vi "automat.vi"() -> ()   [LabVIEW 2014]
uses:
  Timer 2013/Control Timer.ctl
  <vilib>/functionblocks/Edge Detection/One Shot Falling With Input/One Shot Falling With Input.vi
  <vilib>/functionblocks/Edge Detection/One Shot Rising with Input/One Shot Rising with Input.vi
  <vilib>/functionblocks/FB Core/FB Core.xnode
  <vilib>/functionblocks/NI_FunctionBlock Libraries.lvlib
panel:
  out "Center":dbl
  out "Enum 2":T1(ring)
  out "Shutdown":dbl
  out "Left":dbl
  out "Right":dbl
  out "Fault":bool
  out "Right":bool
  out "Center":bool
  out "Left":bool
  in  "Enum":T1(ring)
  out "error out":errorcluster
  in  "error in (no error)":errorcluster
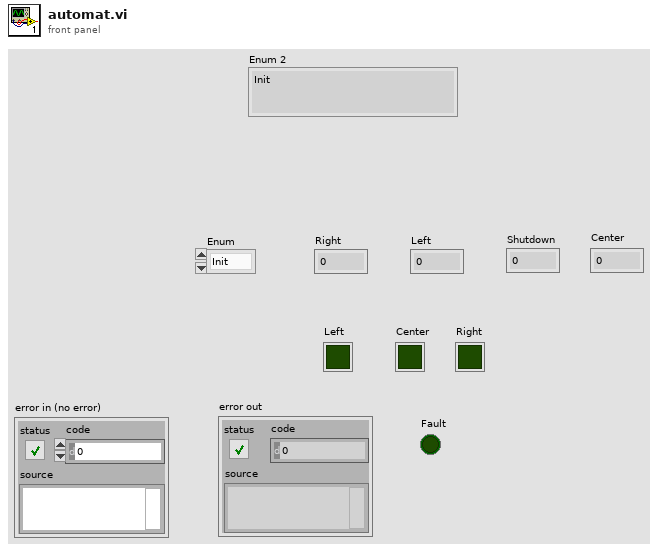
[diagram p1: front panel]
types:
  T1 = enum16{"Init", "Ready", "Shutdown", "Left", "Center", "Right", "Powering up", "Emergency", "Powering down"}
  T2 = typedef "Control Timer.ctl" = enum16{"Timecheck", "Reset"}
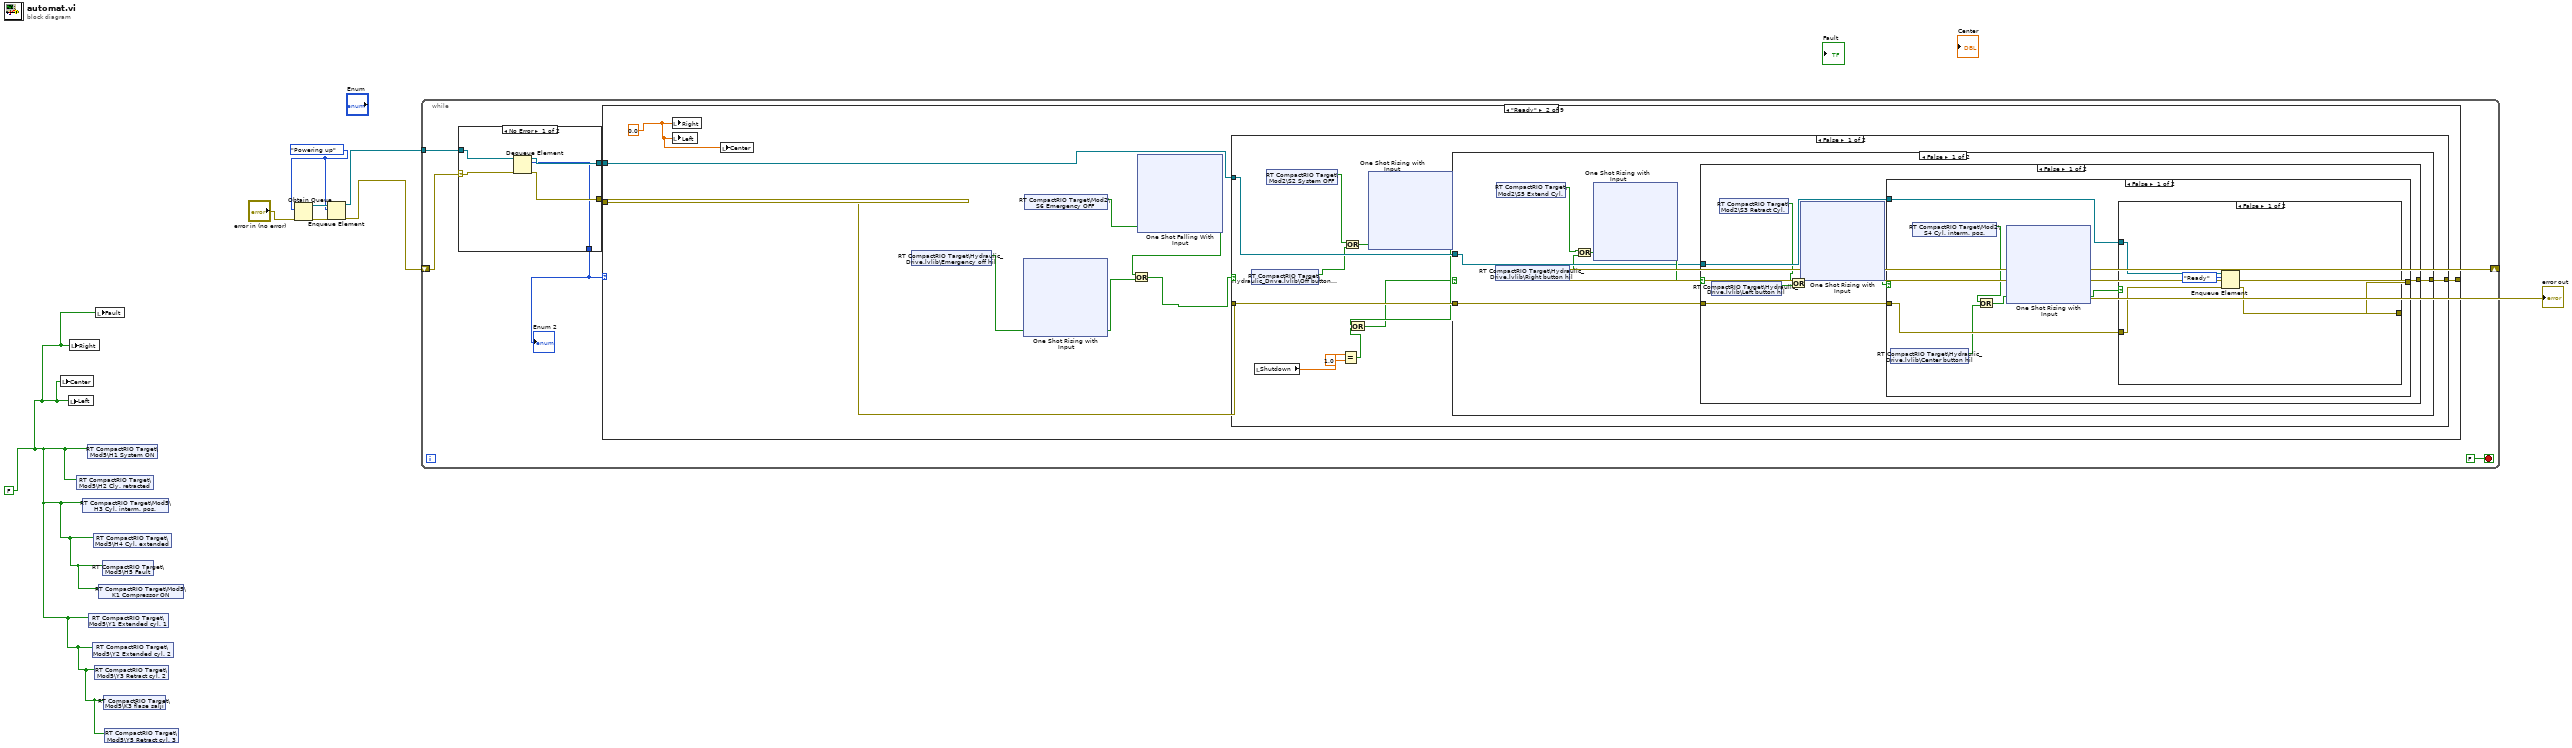
[diagram p0: block diagram]
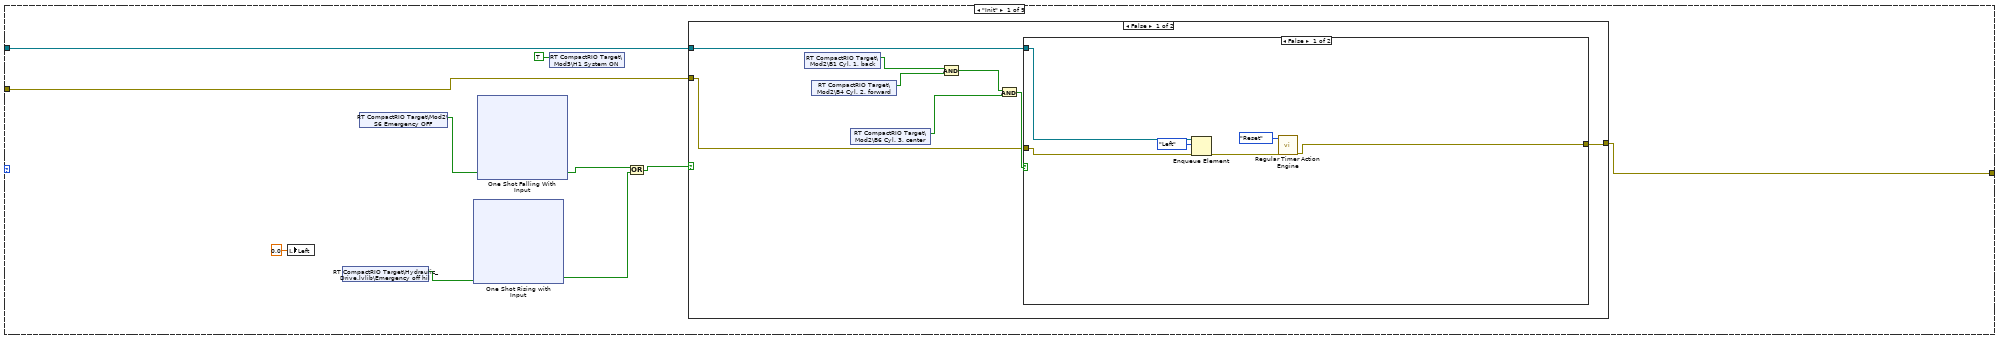
[diagram p2: hidden frame]
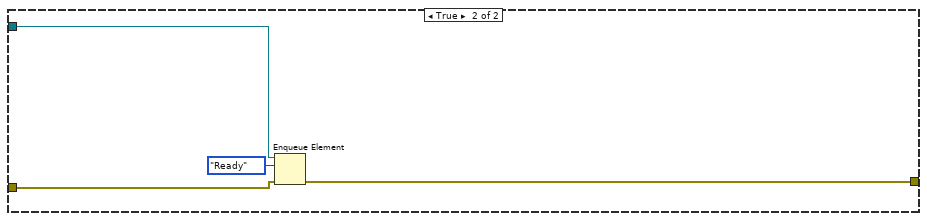
[diagram p3: hidden frame]
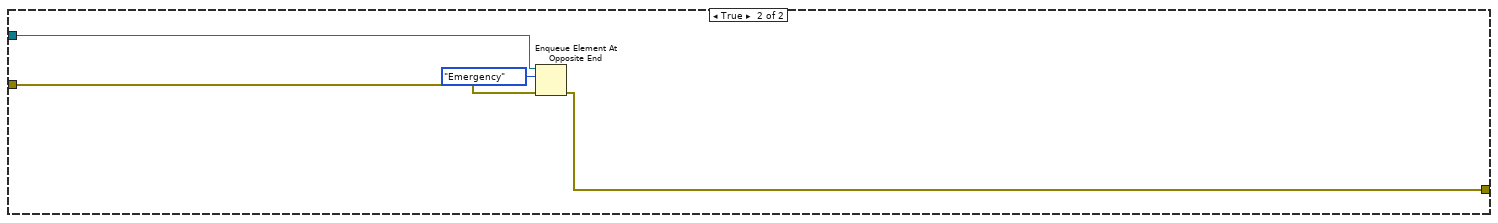
[diagram p4: hidden frame]
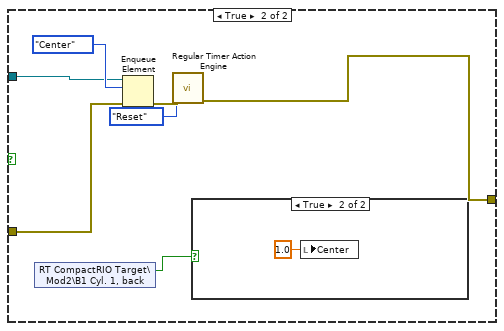
[diagram p5: hidden frame]
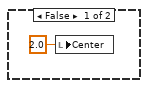
[diagram p6: hidden frame]
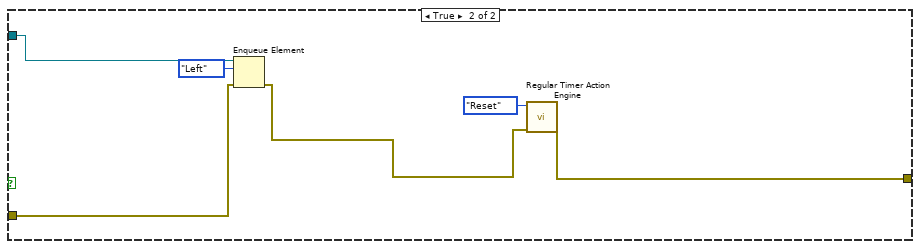
[diagram p7: hidden frame]
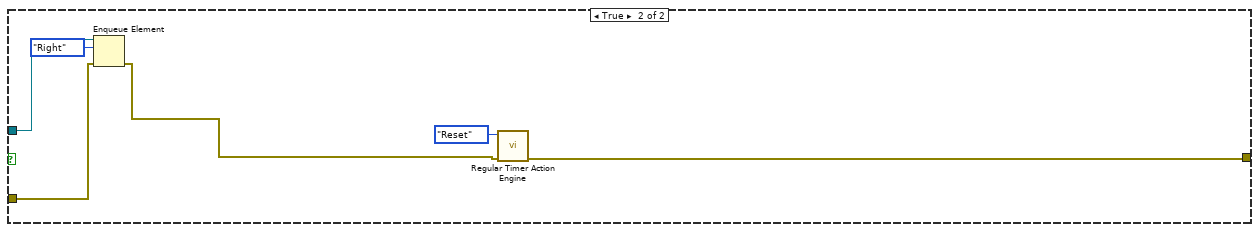
[diagram p8: hidden frame]
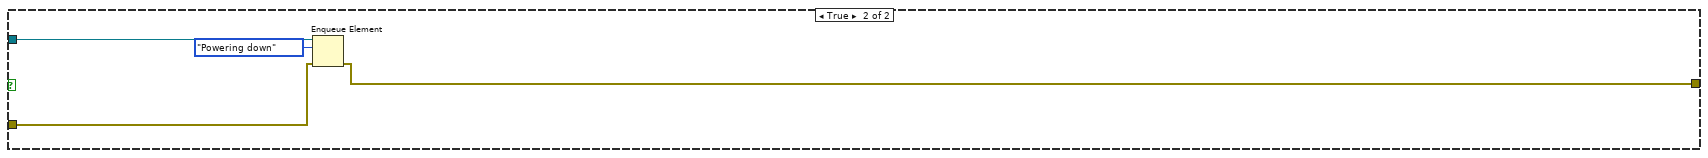
[diagram p9: hidden frame]
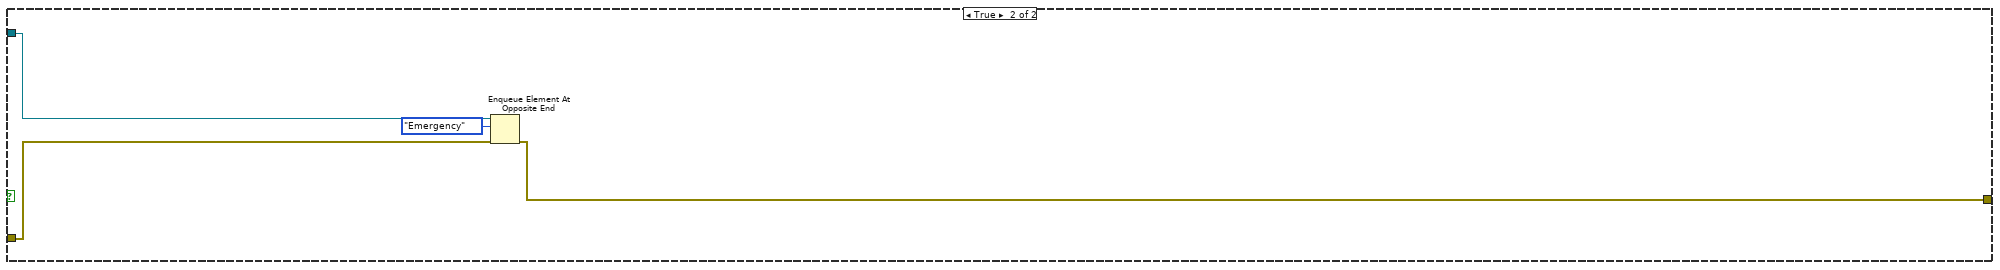
[diagram p10: hidden frame]
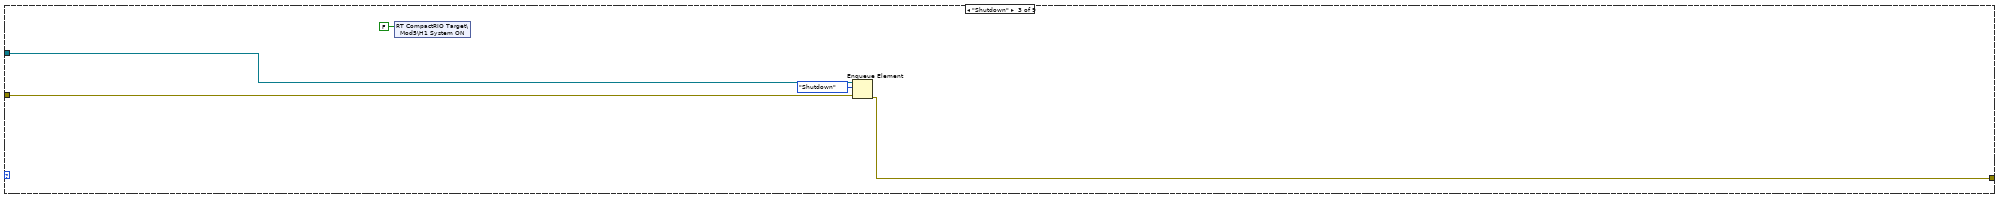
[diagram p11: hidden frame]
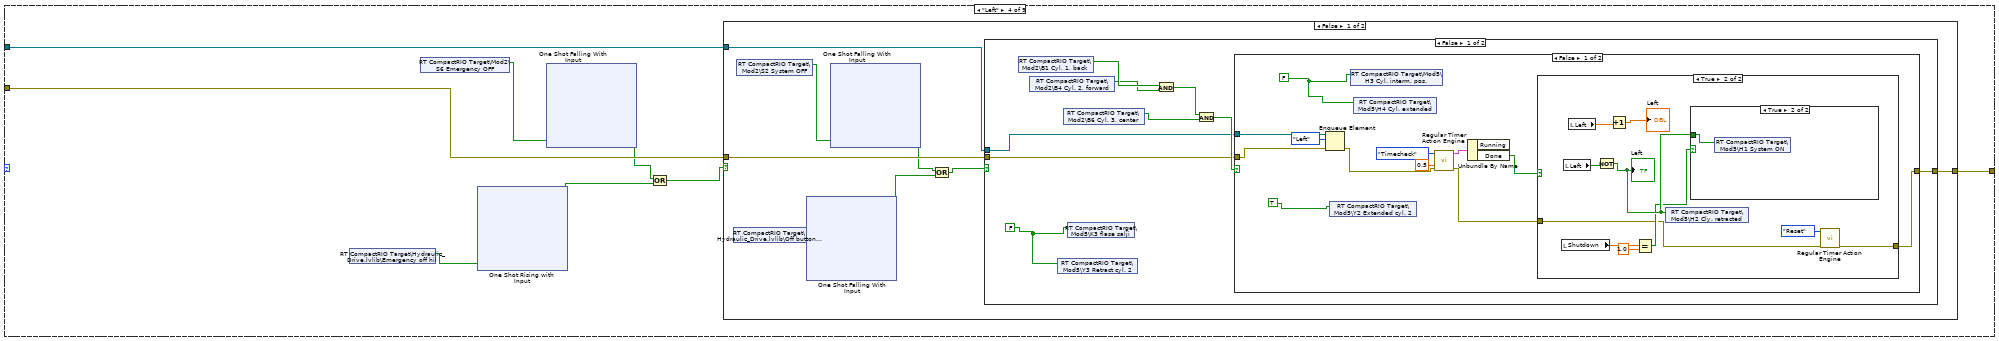
[diagram p12: hidden frame]
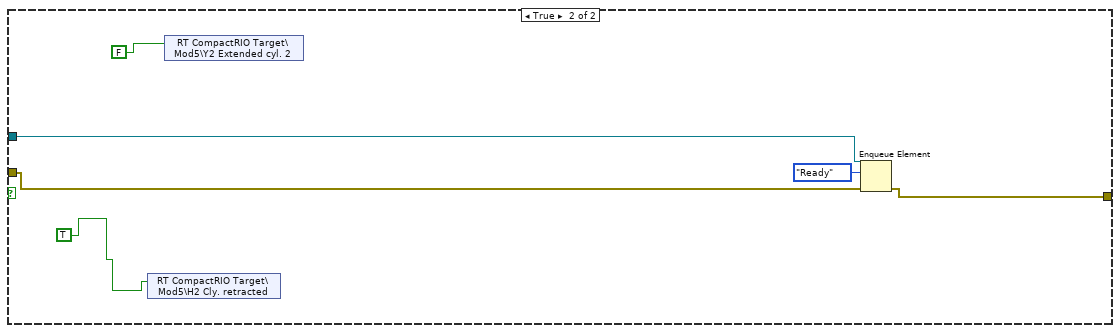
[diagram p15: hidden frame]
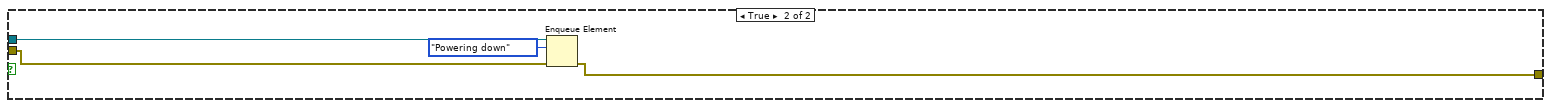
[diagram p16: hidden frame]
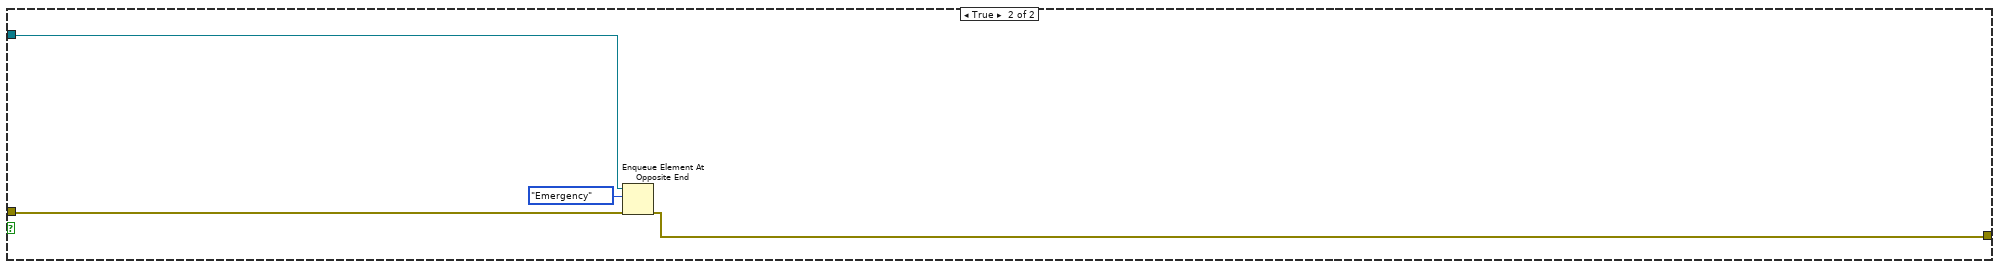
[diagram p17: hidden frame]
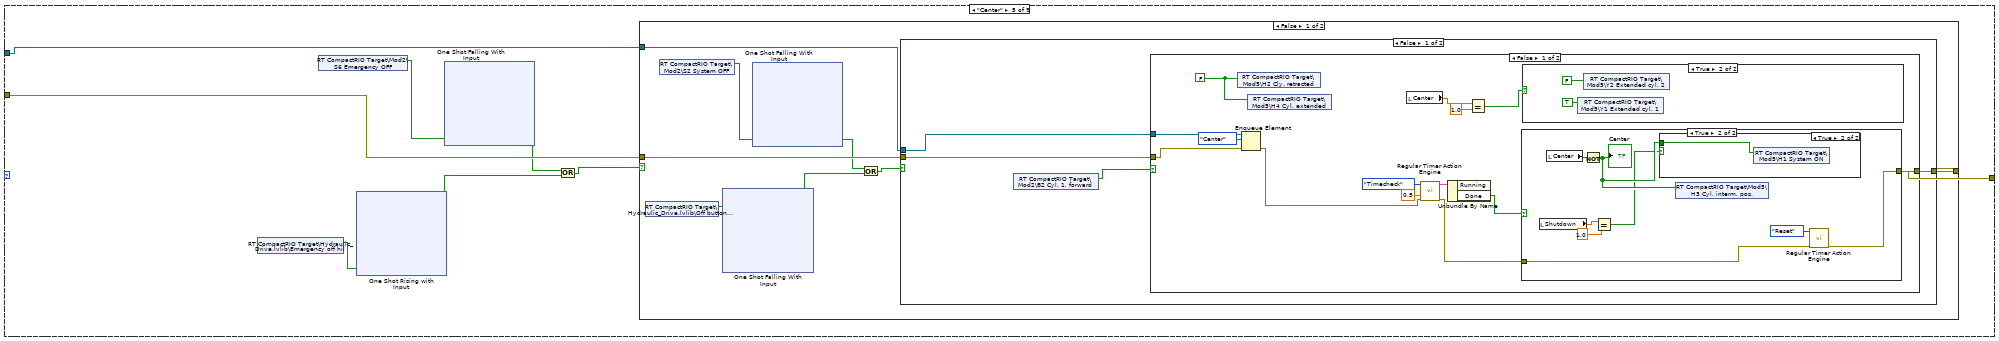
[diagram p18: hidden frame]
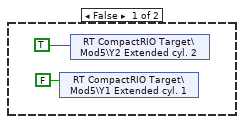
[diagram p19: hidden frame]
diagram:
  w1 = FALSE
  w5 = T1."Powering up" ("Enum")
  n1 = local write "Center"(w1) -> ()
  n2 = local write "Left"(w1) -> ()
  n3 = local write "Right"(w1) -> ()
  n4 = shared-variable "RT CompactRIO Target\\Mod5\\H2 Cly. retracted"(w1) -> ()  [unwired: 1 in, 1 out]
  n5 = shared-variable "RT CompactRIO Target\\Mod5\\H3 Cyl. interm. pos."(w1) -> ()  [unwired: 1 in, 1 out]
  n6 = shared-variable "RT CompactRIO Target\\Mod5\\H1 System ON"(w1) -> ()  [unwired: 1 in, 1 out]
  n7 = shared-variable "RT CompactRIO Target\\Mod5\\Y1 Extended cyl. 1"(w1) -> ()  [unwired: 1 in, 1 out]
  n8 = shared-variable "RT CompactRIO Target\\Mod5\\Y2 Extended cyl. 2"(w1) -> ()  [unwired: 1 in, 1 out]
  n9 = shared-variable "RT CompactRIO Target\\Mod5\\H4 Cyl. extended"(w1) -> ()  [unwired: 1 in, 1 out]
  n10 = shared-variable "RT CompactRIO Target\\Mod5\\Y3 Retract cyl. 2"(w1) -> ()  [unwired: 1 in, 1 out]
  n11 = local write "Fault"(w1) -> ()
  n12 = shared-variable "RT CompactRIO Target\\Mod5\\K1 Compressor ON"(w1) -> ()  [unwired: 1 in, 1 out]
  n13 = shared-variable "RT CompactRIO Target\\Mod5\\H5 Fault"(w1) -> ()  [unwired: 1 in, 1 out]
  n14 = shared-variable "RT CompactRIO Target\\Mod5\\K3 flase salji"(w1) -> ()  [unwired: 1 in, 1 out]
  n15 = shared-variable "RT CompactRIO Target\\Mod5\\Y5 Retract cyl. 3"(w1) -> ()  [unwired: 1 in, 1 out]
  n16 = Obtain Queue(element data type=w5, error in (no error)="error in (no error)") -> (queue out=w6:refnum<queue>, error out=w7:errorcluster)  [unwired: 3 in, 1 out]
  n17 = Enqueue Element(queue=w6, element=w5, error in (no error)=w7) -> (queue out=w4:refnum<queue>, error out=w2:errorcluster)  [unwired: 1 in, 1 out]
  n18 = while {
    tunnel: w4 -> [w15]
    shift-right: [w12] -> w3
    shift-left: w2 -> [w11]
    stop <- FALSE stop-if-true
    n19 = case shown="No Error" w11 {
      selector: w11 -> [w1333 w1336]
      tunnel: w15 -> [w1331 w1335]
      tunnel: [w1332 w1336] -> w13
      tunnel: [w1330 w1335] -> w14
      tunnel: [w1329 T1."Shutdown" ("Enum")] -> w9
      frame No Error {
        n20 = Dequeue Element(queue=w1331, error in (no error)=w1333) -> (queue out=w1330:refnum<queue>, element=w1329:T1, error out=w1332:errorcluster)  [unwired: 1 in, 1 out]
      }
      frame Error {
      }
    }
    "Enum 2" <- w9
    n21 = case shown="\"Ready\"" w9 {
      tunnel: w14 -> [w22 w131 w428 w436 w650 w865 w1080 w1238 w1327]
      tunnel: w13 -> [w23 w132 w429 w437 w651 w866 w1081 w1237 w1328]
      tunnel: [w21 w130 w427 w435 w652 w864 w1079 w1232 w1325] -> w12
      frame "Init" {
        n22 = local write "Left"(0.0 ("Left")) -> ()
        n23 = shared-variable "RT CompactRIO Target\\Hydraulic_Drive.lvlib\\Emergency off hil"() -> (w16:bool)  [unwired: 1 in, 1 out]
        n24 = shared-variable "RT CompactRIO Target\\Mod2\\S6 Emergency OFF"() -> (w24:bool)  [unwired: 1 in, 1 out]
        n25 = xnode "One Shot Rising with Input"("input"=w16) -> ("output"=w17:bool)  [unwired: 1 in, 1 out]
        n26 = xnode "One Shot Falling With Input"("input"=w24) -> ("output"=w18:bool)  [unwired: 1 in, 1 out]
        n27 = shared-variable "RT CompactRIO Target\\Mod5\\H1 System ON"(TRUE ("H1 System ON")) -> ()  [unwired: 1 in, 1 out]
        n28 = Or(x=w18, y=w17) -> (x .or. y?=w19:bool)
        n29 = case shown="False" w19 {
          tunnel: w23 -> [w66 w85]
          tunnel: w22 -> [w64 w84]
          tunnel: [w65 w82] -> w21
          frame False {
            n30 = shared-variable "RT CompactRIO Target\\Mod2\\B1 Cyl. 1, back"() -> (w71:bool)  [unwired: 1 in, 1 out]
            n31 = shared-variable "RT CompactRIO Target\\Mod2\\B4 Cyl. 2, forward"() -> (w70:bool)  [unwired: 1 in, 1 out]
            n32 = shared-variable "RT CompactRIO Target\\Mod2\\B6 Cyl. 3, center"() -> (w68:bool)  [unwired: 1 in, 1 out]
            n33 = And(x=w71, y=w70) -> (x .and. y?=w69:bool)
            n34 = And(x=w69, y=w68) -> (x .and. y?=w67:bool)
            n35 = case shown="False" w67 {
              tunnel: w66 -> [w77 w81]
              tunnel: [w73 w80] -> w65
              tunnel: w64 -> [w76 w79]
              frame False {
                n36 = Enqueue Element(queue=w76, element=T1."Left", error in (no error)=w77) -> (error out=w74:errorcluster)  [unwired: 1 in, 2 out]
                n37 = call "Regular Timer Action Engine.vi"("Enum"=Control_Timer."Reset", "error in"=w74) -> ("error out"=w73:errorcluster)  [unwired: 7 in, 1 out]
              }
              frame True {
                n38 = Enqueue Element(queue=w79, element=T1."Ready", error in (no error)=w81) -> (error out=w80:errorcluster)  [unwired: 1 in, 2 out]
              }
            }
          }
          frame True {
            n39 = Enqueue Element At Opposite End(queue=w84, element=T1."Emergency", error in (no error)=w85) -> (error out=w82:errorcluster)  [unwired: 1 in, 2 out]
          }
        }
      }
      frame "Ready" {
        w125 = 0.0
        n40 = local write "Right"(w125) -> ()
        n41 = local write "Left"(w125) -> ()
        n42 = local write "Center"(w125) -> ()
        n43 = shared-variable "RT CompactRIO Target\\Hydraulic_Drive.lvlib\\Emergency off hil"() -> (w129:bool)  [unwired: 1 in, 1 out]
        n44 = xnode "One Shot Rising with Input"("input"=w129) -> ("output"=w128:bool)  [unwired: 1 in, 1 out]
        n45 = shared-variable "RT CompactRIO Target\\Mod2\\S6 Emergency OFF"() -> (w127:bool)  [unwired: 1 in, 1 out]
        n46 = xnode "One Shot Falling With Input"("input"=w127) -> ("output"=w126:bool)  [unwired: 1 in, 1 out]
        n47 = Or(x=w126, y=w128) -> (x .or. y?=w124:bool)
        n48 = case shown="False" w124 {
          tunnel: w132 -> [w181 w387]
          tunnel: w131 -> [w179 w386]
          tunnel: [w180 w384] -> w130
          frame False {
            n49 = shared-variable "RT CompactRIO Target\\Hydraulic_Drive.lvlib\\Off button hil"() -> (w176:bool)  [unwired: 1 in, 1 out]
            n50 = local read "Shutdown"() -> (w173:dbl)
            n51 = shared-variable "RT CompactRIO Target\\Mod2\\S2 System OFF"() -> (w177:bool)  [unwired: 1 in, 1 out]
            n52 = Equal?(x=w173, y=1.0) -> (x = y?=w175:bool)
            n53 = Or(x=w177, y=w176) -> (x .or. y?=w178:bool)
            n54 = xnode "One Shot Rising with Input"("input"=w178) -> ("output"=w172:bool)  [unwired: 1 in, 1 out]
            n55 = Or(x=w172, y=w175) -> (x .or. y?=w171:bool)
            n56 = case shown="False" w171 {
              tunnel: w181 -> [w225 w383]
              tunnel: [w223 w382] -> w180
              tunnel: w179 -> [w224 w381]
              frame False {
                n57 = shared-variable "RT CompactRIO Target\\Hydraulic_Drive.lvlib\\Right button hil"() -> (w220:bool)  [unwired: 1 in, 1 out]
                n58 = shared-variable "RT CompactRIO Target\\Mod2\\S5 Extend Cyl."() -> (w221:bool)  [unwired: 1 in, 1 out]
                n59 = Or(x=w221, y=w220) -> (x .or. y?=w222:bool)
                n60 = xnode "One Shot Rising with Input"("input"=w222) -> ("output"=w226:bool)  [unwired: 1 in, 1 out]
                n61 = case shown="False" w226 {
                  tunnel: w225 -> [w232 w341]
                  tunnel: w224 -> [w231 w340]
                  tunnel: [w230 w336] -> w223
                  frame False {
                    n62 = shared-variable "RT CompactRIO Target\\Hydraulic_Drive.lvlib\\Left button hil"() -> (w227:bool)  [unwired: 1 in, 1 out]
                    n63 = shared-variable "RT CompactRIO Target\\Mod2\\S3 Retract Cyl."() -> (w228:bool)  [unwired: 1 in, 1 out]
                    n64 = Or(x=w228, y=w227) -> (x .or. y?=w229:bool)
                    n65 = xnode "One Shot Rising with Input"("input"=w229) -> ("output"=w233:bool)  [unwired: 1 in, 1 out]
                    n66 = case shown="False" w233 {
                      tunnel: w232 -> [w239 w296]
                      tunnel: w231 -> [w238 w295]
                      tunnel: [w237 w293] -> w230
                      frame False {
                        n67 = shared-variable "RT CompactRIO Target\\Hydraulic_Drive.lvlib\\Center button hil"() -> (w234:bool)  [unwired: 1 in, 1 out]
                        n68 = shared-variable "RT CompactRIO Target\\Mod2\\S4 Cyl. interm. pos."() -> (w236:bool)  [unwired: 1 in, 1 out]
                        n69 = Or(x=w236, y=w234) -> (x .or. y?=w235:bool)
                        n70 = xnode "One Shot Rising with Input"("input"=w235) -> ("output"=w240:bool)  [unwired: 1 in, 1 out]
                        n71 = case shown="False" w240 {
                          tunnel: w239 -> [w244 w250]
                          tunnel: w238 -> [w242 w249]
                          tunnel: [w243 w247] -> w237
                          frame False {
                            n72 = Enqueue Element(queue=w242, element=T1."Ready", error in (no error)=w244) -> (error out=w243:errorcluster)  [unwired: 1 in, 2 out]
                          }
                          frame True {
                            n73 = shared-variable "RT CompactRIO Target\\Mod2\\B1 Cyl. 1, back"() -> (w245:bool)  [unwired: 1 in, 1 out]
                            n74 = Enqueue Element(queue=w249, element=T1."Center", error in (no error)=w250) -> (error out=w248:errorcluster)  [unwired: 1 in, 2 out]
                            n75 = call "Regular Timer Action Engine.vi"("Enum"=Control_Timer."Reset", "error in"=w248) -> ("error out"=w247:errorcluster)  [unwired: 7 in, 1 out]
                            n76 = case shown="True" w245 {
                              frame False {
                                n77 = local write "Center"(2.0 ("Center")) -> ()
                              }
                              frame True {
                                n78 = local write "Center"(1.0 ("Center")) -> ()
                              }
                            }
                          }
                        }
                      }
                      frame True {
                        n79 = Enqueue Element(queue=w295, element=T1."Left", error in (no error)=w296) -> (error out=w294:errorcluster)  [unwired: 1 in, 2 out]
                        n80 = call "Regular Timer Action Engine.vi"("Enum"=Control_Timer."Reset", "error in"=w294) -> ("error out"=w293:errorcluster)  [unwired: 7 in, 1 out]
                      }
                    }
                  }
                  frame True {
                    n81 = Enqueue Element(queue=w340, element=T1."Right", error in (no error)=w341) -> (error out=w338:errorcluster)  [unwired: 1 in, 2 out]
                    n82 = call "Regular Timer Action Engine.vi"("Enum"=Control_Timer."Reset", "error in"=w338) -> ("error out"=w336:errorcluster)  [unwired: 7 in, 1 out]
                  }
                }
              }
              frame True {
                n83 = Enqueue Element(queue=w381, element=T1."Powering down", error in (no error)=w383) -> (error out=w382:errorcluster)  [unwired: 1 in, 2 out]
              }
            }
          }
          frame True {
            n84 = Enqueue Element At Opposite End(queue=w386, element=T1."Emergency", error in (no error)=w387) -> (error out=w384:errorcluster)  [unwired: 1 in, 2 out]
          }
        }
      }
      frame "Shutdown" {
        n85 = shared-variable "RT CompactRIO Target\\Mod5\\H1 System ON"(FALSE ("H1 System ON")) -> ()  [unwired: 1 in, 1 out]
        n86 = Enqueue Element(queue=w428, element=T1."Shutdown", error in (no error)=w429) -> (error out=w427:errorcluster)  [unwired: 1 in, 2 out]
      }
      frame "Left" {
        n87 = shared-variable "RT CompactRIO Target\\Hydraulic_Drive.lvlib\\Emergency off hil"() -> (w432:bool)  [unwired: 1 in, 1 out]
        n88 = shared-variable "RT CompactRIO Target\\Mod2\\S6 Emergency OFF"() -> (w438:bool)  [unwired: 1 in, 1 out]
        n89 = xnode "One Shot Rising with Input"("input"=w432) -> ("output"=w431:bool)  [unwired: 1 in, 1 out]
        n90 = xnode "One Shot Falling With Input"("input"=w438) -> ("output"=w433:bool)  [unwired: 1 in, 1 out]
        n91 = Or(x=w433, y=w431) -> (x .or. y?=w434:bool)
        n92 = case shown="False" w434 {
          tunnel: w437 -> [w483 w607]
          tunnel: w436 -> [w482 w606]
          tunnel: [w481 w604] -> w435
          frame False {
            n93 = shared-variable "RT CompactRIO Target\\Hydraulic_Drive.lvlib\\Off button hil"() -> (w477:bool)  [unwired: 1 in, 1 out]
            n94 = shared-variable "RT CompactRIO Target\\Mod2\\S2 System OFF"() -> (w484:bool)  [unwired: 1 in, 1 out]
            n95 = xnode "One Shot Falling With Input"("input"=w477) -> ("output"=w478:bool)  [unwired: 1 in, 1 out]
            n96 = xnode "One Shot Falling With Input"("input"=w484) -> ("output"=w479:bool)  [unwired: 1 in, 1 out]
            n97 = Or(x=w479, y=w478) -> (x .or. y?=w480:bool)
            n98 = case shown="False" w480 {
              tunnel: w483 -> [w529 w565]
              tunnel: w482 -> [w527 w564]
              tunnel: [w528 w562] -> w481
              frame False {
                w523 = FALSE
                n99 = shared-variable "RT CompactRIO Target\\Mod2\\B1 Cyl. 1, back"() -> (w525:bool)  [unwired: 1 in, 1 out]
                n100 = shared-variable "RT CompactRIO Target\\Mod2\\B4 Cyl. 2, forward"() -> (w524:bool)  [unwired: 1 in, 1 out]
                n101 = shared-variable "RT CompactRIO Target\\Mod5\\Y3 Retract cyl. 2"(w523) -> ()  [unwired: 1 in, 1 out]
                n102 = shared-variable "RT CompactRIO Target\\Mod2\\B6 Cyl. 3, center"() -> (w526:bool)  [unwired: 1 in, 1 out]
                n103 = shared-variable "RT CompactRIO Target\\Mod5\\K3 flase salji"(w523) -> ()  [unwired: 1 in, 1 out]
                n104 = And(x=w525, y=w524) -> (x .and. y?=w531:bool)
                n105 = And(x=w531, y=w526) -> (x .and. y?=w530:bool)
                n106 = case shown="False" w530 {
                  tunnel: w529 -> [w543 w561]
                  tunnel: [w533 w560] -> w528
                  tunnel: w527 -> [w542 w559]
                  frame False {
                    w540 = FALSE
                    n107 = Enqueue Element(queue=w542, element=T1."Left", error in (no error)=w543) -> (error out=w539:errorcluster)  [unwired: 1 in, 2 out]
                    n108 = shared-variable "RT CompactRIO Target\\Mod5\\Y2 Extended cyl. 2"(TRUE) -> ()  [unwired: 1 in, 1 out]
                    n109 = shared-variable "RT CompactRIO Target\\Mod5\\H3 Cyl. interm. pos."(w540) -> ()  [unwired: 1 in, 1 out]
                    n110 = shared-variable "RT CompactRIO Target\\Mod5\\H4 Cyl. extended"(w540) -> ()  [unwired: 1 in, 1 out]
                    n111 = call "Regular Timer Action Engine.vi"("Enum"=Control_Timer."Timecheck", "Time Target"=0.5, "error in"=w539) -> ("Status"=w536:cluster{"Running":bool, "Done":bool}, "error out"=w534:errorcluster)  [unwired: 6 in]
                    n112 = Unbundle By Name(w536) -> ("Done"=w535:bool)  [unwired: 1 out]
                    n113 = case shown="True" w535 {
                      tunnel: w534 -> [w544 w547]
                      tunnel: [w544 w546] -> w533
                      frame False {
                      }
                      frame True {
                        n114 = local read "Shutdown"() -> (w549:dbl)
                        n115 = local read "Left"() -> (w552:bool)
                        n116 = local read "Left"() -> (w554:dbl)
                        n117 = Not(x=w552) -> (.not. x?=w551:bool)
                        "Left" <- w551
                        n118 = Increment(x=w554) -> (x+1=→"Left":dbl)
                        n119 = Equal?(x=w549, y=1.0) -> (x = y?=w550:bool)
                        n120 = shared-variable "RT CompactRIO Target\\Mod5\\H2 Cly. retracted"(w551) -> ()  [unwired: 1 in, 1 out]
                        n121 = case shown="True" w550 {
                          tunnel: w551 -> [_ w555]
                          frame False {
                          }
                          frame True {
                            n122 = shared-variable "RT CompactRIO Target\\Mod5\\H1 System ON"(w555) -> ()  [unwired: 1 in, 1 out]
                          }
                        }
                        n123 = call "Regular Timer Action Engine.vi"("Enum"=Control_Timer."Reset", "error in"=w547) -> ("error out"=w546:errorcluster)  [unwired: 7 in, 1 out]
                      }
                    }
                  }
                  frame True {
                    n124 = shared-variable "RT CompactRIO Target\\Mod5\\H2 Cly. retracted"(TRUE) -> ()  [unwired: 1 in, 1 out]
                    n125 = shared-variable "RT CompactRIO Target\\Mod5\\Y2 Extended cyl. 2"(FALSE ("K1 Compressor ON")) -> ()  [unwired: 1 in, 1 out]
                    n126 = Enqueue Element(queue=w559, element=T1."Ready", error in (no error)=w561) -> (error out=w560:errorcluster)  [unwired: 1 in, 2 out]
                  }
                }
              }
              frame True {
                n127 = Enqueue Element(queue=w564, element=T1."Powering down", error in (no error)=w565) -> (error out=w562:errorcluster)  [unwired: 1 in, 2 out]
              }
            }
          }
          frame True {
            n128 = Enqueue Element At Opposite End(queue=w606, element=T1."Emergency", error in (no error)=w607) -> (error out=w604:errorcluster)  [unwired: 1 in, 2 out]
          }
        }
      }
      frame "Center" {
        n129 = shared-variable "RT CompactRIO Target\\Hydraulic_Drive.lvlib\\Emergency off hil"() -> (w646:bool)  [unwired: 1 in, 1 out]
        n130 = shared-variable "RT CompactRIO Target\\Mod2\\S6 Emergency OFF"() -> (w653:bool)  [unwired: 1 in, 1 out]
        n131 = xnode "One Shot Rising with Input"("input"=w646) -> ("output"=w647:bool)  [unwired: 1 in, 1 out]
        n132 = xnode "One Shot Falling With Input"("input"=w653) -> ("output"=w648:bool)  [unwired: 1 in, 1 out]
        n133 = Or(x=w648, y=w647) -> (x .or. y?=w649:bool)
        n134 = case shown="False" w649 {
          tunnel: w651 -> [w698 w821]
          tunnel: w650 -> [w697 w820]
          tunnel: [w696 w818] -> w652
          frame False {
            n135 = shared-variable "RT CompactRIO Target\\Hydraulic_Drive.lvlib\\Off button hil"() -> (w692:bool)  [unwired: 1 in, 1 out]
            n136 = shared-variable "RT CompactRIO Target\\Mod2\\S2 System OFF"() -> (w699:bool)  [unwired: 1 in, 1 out]
            n137 = xnode "One Shot Falling With Input"("input"=w692) -> ("output"=w693:bool)  [unwired: 1 in, 1 out]
            n138 = xnode "One Shot Falling With Input"("input"=w699) -> ("output"=w694:bool)  [unwired: 1 in, 1 out]
            n139 = Or(x=w694, y=w693) -> (x .or. y?=w695:bool)
            n140 = case shown="False" w695 {
              tunnel: w698 -> [w741 w779]
              tunnel: w697 -> [w739 w778]
              tunnel: [w740 w776] -> w696
              frame False {
                n141 = shared-variable "RT CompactRIO Target\\Mod2\\B2 Cyl. 1, forward"() -> (w738:bool)  [unwired: 1 in, 1 out]
                n142 = case shown="False" w738 {
                  tunnel: w741 -> [w755 w775]
                  tunnel: [w745 w774] -> w740
                  tunnel: w739 -> [w754 w773]
                  frame False {
                    w752 = FALSE
                    n143 = shared-variable "RT CompactRIO Target\\Mod5\\H2 Cly. retracted"(w752) -> ()  [unwired: 1 in, 1 out]
                    n144 = Enqueue Element(queue=w754, element=T1."Center", error in (no error)=w755) -> (error out=w751:errorcluster)  [unwired: 1 in, 2 out]
                    n145 = shared-variable "RT CompactRIO Target\\Mod5\\H4 Cyl. extended"(w752) -> ()  [unwired: 1 in, 1 out]
                    n146 = local read "Center"() -> (w743:dbl)
                    n147 = call "Regular Timer Action Engine.vi"("Enum"=Control_Timer."Timecheck", "Time Target"=0.5, "error in"=w751) -> ("Status"=w748:cluster{"Running":bool, "Done":bool}, "error out"=w746:errorcluster)  [unwired: 6 in]
                    n148 = Unbundle By Name(w748) -> ("Done"=w747:bool)  [unwired: 1 out]
                    n149 = Equal?(x=w743, y=1.0) -> (x = y?=w744:bool)
                    n150 = case shown="True" w747 {
                      tunnel: w746 -> [w760 w767]
                      tunnel: [w760 w766] -> w745
                      frame False {
                      }
                      frame True {
                        n151 = local read "Shutdown"() -> (w762:dbl)
                        n152 = local read "Center"() -> (w768:bool)
                        n153 = Not(x=w768) -> (.not. x?=w764:bool)
                        "Center" <- w764
                        n154 = Equal?(x=w762, y=1.0) -> (x = y?=w763:bool)
                        n155 = case shown="True" w763 {
                          tunnel: w764 -> [_ w769]
                          frame False {
                          }
                          frame True {
                            n156 = shared-variable "RT CompactRIO Target\\Mod5\\H1 System ON"(w769) -> ()  [unwired: 1 in, 1 out]
                          }
                        }
                        n157 = shared-variable "RT CompactRIO Target\\Mod5\\H3 Cyl. interm. pos."(w764) -> ()  [unwired: 1 in, 1 out]
                        n158 = call "Regular Timer Action Engine.vi"("Enum"=Control_Timer."Reset", "error in"=w767) -> ("error out"=w766:errorcluster)  [unwired: 7 in, 1 out]
                      }
                    }
                    n159 = case shown="True" w744 {
                      frame False {
                        n160 = shared-variable "RT CompactRIO Target\\Mod5\\Y1 Extended cyl. 1"(FALSE ("Y1 Extended cyl. 1")) -> ()  [unwired: 1 in, 1 out]
                        n161 = shared-variable "RT CompactRIO Target\\Mod5\\Y2 Extended cyl. 2"(TRUE ("K1 Compressor ON")) -> ()  [unwired: 1 in, 1 out]
                      }
                      frame True {
                        n162 = shared-variable "RT CompactRIO Target\\Mod5\\Y1 Extended cyl. 1"(TRUE ("Y1 Extended cyl. 1")) -> ()  [unwired: 1 in, 1 out]
                        n163 = shared-variable "RT CompactRIO Target\\Mod5\\Y2 Extended cyl. 2"(FALSE ("K1 Compressor ON")) -> ()  [unwired: 1 in, 1 out]
                      }
                    }
                  }
                  frame True {
                    w770 = FALSE ("K1 Compressor ON")
                    n164 = shared-variable "RT CompactRIO Target\\Mod5\\H3 Cyl. interm. pos."(TRUE) -> ()  [unwired: 1 in, 1 out]
                    n165 = shared-variable "RT CompactRIO Target\\Mod5\\Y1 Extended cyl. 1"(w770) -> ()  [unwired: 1 in, 1 out]
                    n166 = shared-variable "RT CompactRIO Target\\Mod5\\Y2 Extended cyl. 2"(w770) -> ()  [unwired: 1 in, 1 out]
                    n167 = Enqueue Element(queue=w773, element=T1."Ready", error in (no error)=w775) -> (error out=w774:errorcluster)  [unwired: 1 in, 2 out]
                  }
                }
              }
              frame True {
                n168 = Enqueue Element(queue=w778, element=T1."Powering down", error in (no error)=w779) -> (error out=w776:errorcluster)  [unwired: 1 in, 2 out]
              }
            }
          }
          frame True {
            n169 = Enqueue Element At Opposite End(queue=w820, element=T1."Emergency", error in (no error)=w821) -> (error out=w818:errorcluster)  [unwired: 1 in, 2 out]
          }
        }
      }
      frame "Right" {
        n170 = shared-variable "RT CompactRIO Target\\Hydraulic_Drive.lvlib\\Emergency off hil"() -> (w860:bool)  [unwired: 1 in, 1 out]
        n171 = shared-variable "RT CompactRIO Target\\Mod2\\S6 Emergency OFF"() -> (w867:bool)  [unwired: 1 in, 1 out]
        n172 = xnode "One Shot Rising with Input"("input"=w860) -> ("output"=w861:bool)  [unwired: 1 in, 1 out]
        n173 = xnode "One Shot Falling With Input"("input"=w867) -> ("output"=w862:bool)  [unwired: 1 in, 1 out]
        n174 = Or(x=w862, y=w861) -> (x .or. y?=w863:bool)
        n175 = case shown="False" w863 {
          tunnel: w866 -> [w912 w1036]
          tunnel: w865 -> [w911 w1035]
          tunnel: [w910 w1033] -> w864
          frame False {
            n176 = shared-variable "RT CompactRIO Target\\Mod2\\S2 System OFF"() -> (w913:bool)  [unwired: 1 in, 1 out]
            n177 = shared-variable "RT CompactRIO Target\\Hydraulic_Drive.lvlib\\Off button hil"() -> (w906:bool)  [unwired: 1 in, 1 out]
            n178 = xnode "One Shot Falling With Input"("input"=w906) -> ("output"=w907:bool)  [unwired: 1 in, 1 out]
            n179 = xnode "One Shot Falling With Input"("input"=w913) -> ("output"=w908:bool)  [unwired: 1 in, 1 out]
            n180 = Or(x=w908, y=w907) -> (x .or. y?=w909:bool)
            n181 = case shown="True" w909 {
              tunnel: w912 -> [w957 w994]
              tunnel: w911 -> [w955 w993]
              tunnel: [w956 w991] -> w910
              frame False {
                n182 = shared-variable "RT CompactRIO Target\\Mod2\\B7 Cyl. 3, forward"() -> (w953:bool)  [unwired: 1 in, 1 out]
                n183 = shared-variable "RT CompactRIO Target\\Mod2\\B3 Cyl. 2, back"() -> (w954:bool)  [unwired: 1 in, 1 out]
                n184 = shared-variable "RT CompactRIO Target\\Mod2\\B5 Cyl. 3, back"() -> (w952:bool)  [unwired: 1 in, 1 out]
                n185 = And(x=w954, y=w953) -> (x .and. y?=w959:bool)
                n186 = And(x=w959, y=w952) -> (x .and. y?=w958:bool)
                n187 = case shown="True" w958 {
                  tunnel: w957 -> [w971 w989]
                  tunnel: [w961 w988] -> w956
                  tunnel: w955 -> [w970 w987]
                  frame False {
                    w960 = TRUE ("K3 flase salji")
                    w968 = FALSE
                    n188 = shared-variable "RT CompactRIO Target\\Mod5\\H3 Cyl. interm. pos."(w968) -> ()  [unwired: 1 in, 1 out]
                    n189 = shared-variable "RT CompactRIO Target\\Mod5\\H2 Cly. retracted"(w968) -> ()  [unwired: 1 in, 1 out]
                    n190 = Enqueue Element(queue=w970, element=T1."Right", error in (no error)=w971) -> (error out=w967:errorcluster)  [unwired: 1 in, 2 out]
                    n191 = shared-variable "RT CompactRIO Target\\Mod5\\K3 flase salji"(w960) -> ()  [unwired: 1 in, 1 out]
                    n192 = shared-variable "RT CompactRIO Target\\Mod5\\Y1 Extended cyl. 1"(w960) -> ()  [unwired: 1 in, 1 out]
                    n193 = shared-variable "RT CompactRIO Target\\Mod5\\Y3 Retract cyl. 2"(w960) -> ()  [unwired: 1 in, 1 out]
                    n194 = call "Regular Timer Action Engine.vi"("Enum"=Control_Timer."Timecheck", "Time Target"=0.5, "error in"=w967) -> ("Status"=w964:cluster{"Running":bool, "Done":bool}, "error out"=w962:errorcluster)  [unwired: 6 in]
                    n195 = Unbundle By Name(w964) -> ("Done"=w963:bool)  [unwired: 1 out]
                    n196 = case shown="True" w963 {
                      tunnel: w962 -> [w972 w982]
                      tunnel: [w972 w981] -> w961
                      frame False {
                      }
                      frame True {
                        n197 = local read "Right"() -> (w979:dbl)
                        n198 = local read "Right"() -> (w977:bool)
                        n199 = local read "Shutdown"() -> (w975:dbl)
                        n200 = Increment(x=w979) -> (x+1=→"Right":dbl)
                        n201 = Not(x=w977) -> (.not. x?=w973:bool)
                        "Right" <- w973
                        n202 = Equal?(x=w975, y=1.0) -> (x = y?=w976:bool)
                        n203 = case shown="False" w976 {
                          tunnel: w973 -> [_ w983]
                          frame False {
                          }
                          frame True {
                            n204 = shared-variable "RT CompactRIO Target\\Mod5\\H1 System ON"(w983) -> ()  [unwired: 1 in, 1 out]
                          }
                        }
                        n205 = shared-variable "RT CompactRIO Target\\Mod5\\H4 Cyl. extended"(w973) -> ()  [unwired: 1 in, 1 out]
                        n206 = call "Regular Timer Action Engine.vi"("Enum"=Control_Timer."Reset", "error in"=w982) -> ("error out"=w981:errorcluster)  [unwired: 7 in, 1 out]
                      }
                    }
                  }
                  frame True {
                    w984 = TRUE
                    n207 = shared-variable "RT CompactRIO Target\\Mod5\\H4 Cyl. extended"(w984) -> ()  [unwired: 1 in, 1 out]
                    n208 = shared-variable "RT CompactRIO Target\\Mod5\\Y3 Retract cyl. 2"(w984) -> ()  [unwired: 1 in, 1 out]
                    n209 = shared-variable "RT CompactRIO Target\\Mod5\\Y1 Extended cyl. 1"(FALSE ("K1 Compressor ON")) -> ()  [unwired: 1 in, 1 out]
                    n210 = shared-variable "RT CompactRIO Target\\Mod5\\K3 flase salji"(w984) -> ()  [unwired: 1 in, 1 out]
                    n211 = Enqueue Element(queue=w987, element=T1."Ready", error in (no error)=w989) -> (error out=w988:errorcluster)  [unwired: 1 in, 2 out]
                  }
                }
              }
              frame True {
                n212 = Enqueue Element(queue=w993, element=T1."Powering down", error in (no error)=w994) -> (error out=w991:errorcluster)  [unwired: 1 in, 2 out]
                n213 = local write "Shutdown"(1.0 ("Shutdown")) -> ()
              }
            }
          }
          frame True {
            n214 = Enqueue Element At Opposite End(queue=w1035, element=T1."Emergency", error in (no error)=w1036) -> (error out=w1033:errorcluster)  [unwired: 1 in, 2 out]
          }
        }
      }
      frame "Powering up", Default {
        n215 = shared-variable "RT CompactRIO Target\\Mod2\\S6 Emergency OFF"() -> (w1082:bool)  [unwired: 1 in, 1 out]
        n216 = shared-variable "RT CompactRIO Target\\Mod5\\H1 System ON"(FALSE ("H1 System ON")) -> ()  [unwired: 1 in, 1 out]
        n217 = shared-variable "RT CompactRIO Target\\Hydraulic_Drive.lvlib\\Emergency off hil"() -> (w1075:bool)  [unwired: 1 in, 1 out]
        n218 = xnode "One Shot Falling With Input"("input"=w1082) -> ("output"=w1076:bool)  [unwired: 1 in, 1 out]
        n219 = Or(x=w1076, y=w1075) -> (x .or. y?=w1077:bool)
        n220 = case shown="False" w1077 {
          tunnel: w1081 -> [w1090 w1188]
          tunnel: w1080 -> [w1089 w1187]
          tunnel: [w1088 w1185] -> w1079
          frame False {
            n221 = shared-variable "RT CompactRIO Target\\Mod2\\S1 System ON"() -> (w1091:bool)  [unwired: 1 in, 1 out]
            n222 = shared-variable "RT CompactRIO Target\\Hydraulic_Drive.lvlib\\On button hil"() -> (w1085:bool)  [unwired: 1 in, 1 out]
            n223 = xnode "One Shot Rising with Input"("input"=w1085) -> ("output"=w1084:bool)  [unwired: 1 in, 1 out]
            n224 = xnode "One Shot Rising with Input"("input"=w1091) -> ("output"=w1087:bool)  [unwired: 1 in, 1 out]
            n225 = Or(x=w1087, y=w1084) -> (x .or. y?=w1086:bool)
            n226 = case shown="True" w1086 {
              tunnel: w1090 -> [w1133 w1135]
              tunnel: w1089 -> [w1131 w1136]
              tunnel: [w1132 w1134] -> w1088
              frame False {
                n227 = Enqueue Element(queue=w1131, element=T1."Powering up", error in (no error)=w1133) -> (error out=w1132:errorcluster)  [unwired: 1 in, 2 out]
              }
              frame True {
                n228 = shared-variable "RT CompactRIO Target\\Mod5\\H5 Fault"() -> (w1137:bool)  [unwired: 1 in, 1 out]
                n229 = case shown="False" w1137 {
                  tunnel: w1136 -> [w1139 w1145]
                  tunnel: w1135 -> [w1141 w1146]
                  tunnel: [w1140 w1143] -> w1134
                  frame False {
                    n230 = Enqueue Element(queue=w1139, element=T1."Init", error in (no error)=w1141) -> (error out=w1140:errorcluster)  [unwired: 1 in, 2 out]
                  }
                  frame True {
                    w1142 = FALSE ("H5 Fault")
                    n231 = Enqueue Element(queue=w1145, element=T1."Powering up", error in (no error)=w1146) -> (error out=w1143:errorcluster)  [unwired: 1 in, 2 out]
                    n232 = shared-variable "RT CompactRIO Target\\Mod5\\H5 Fault"(w1142) -> ()  [unwired: 1 in, 1 out]
                    n233 = local write "Fault"(w1142) -> ()
                  }
                }
              }
            }
          }
          frame True {
            n234 = Enqueue Element At Opposite End(queue=w1187, element=T1."Emergency", error in (no error)=w1188) -> (error out=w1185:errorcluster)  [unwired: 1 in, 2 out]
          }
        }
        "Shutdown" <- 0.0 ("Shutdown")
      }
      frame "Emergency" {
        w1227 = FALSE
        n235 = Flush Queue(queue=w1238, error in (no error)=w1237) -> (queue out=w1233:refnum<queue>, error out=w1234:errorcluster)  [unwired: 1 out]
        n236 = shared-variable "RT CompactRIO Target\\Mod5\\H5 Fault"(TRUE ("H5 Fault")) -> ()  [unwired: 1 in, 1 out]
        n237 = shared-variable "RT CompactRIO Target\\Mod5\\Y3 Retract cyl. 2"(w1227) -> ()  [unwired: 1 in, 1 out]
        n238 = shared-variable "RT CompactRIO Target\\Mod5\\Y1 Extended cyl. 1"(w1227) -> ()  [unwired: 1 in, 1 out]
        n239 = shared-variable "RT CompactRIO Target\\Mod5\\Y2 Extended cyl. 2"(w1227) -> ()  [unwired: 1 in, 1 out]
        n240 = shared-variable "RT CompactRIO Target\\Mod5\\K3 flase salji"(w1227) -> ()  [unwired: 1 in, 1 out]
        n241 = shared-variable "RT CompactRIO Target\\Mod2\\S6 Emergency OFF"() -> (w1235:bool)  [unwired: 1 in, 1 out]
        n242 = shared-variable "RT CompactRIO Target\\Hydraulic_Drive.lvlib\\Emergency off hil"() -> (w1229:bool)  [unwired: 1 in, 1 out]
        n243 = xnode "One Shot Falling With Input"("input"=w1235) -> ("output"=w1230:bool)  [unwired: 1 in, 1 out]
        n244 = xnode "One Shot Rising with Input"("input"=w1229) -> ("output"=w1228:bool)  [unwired: 1 in, 1 out]
        n245 = Or(x=w1230, y=w1228) -> (x .or. y?=w1231:bool)
        n246 = case shown="False" w1231 {
          tunnel: w1234 -> [w1280 w1284]
          tunnel: w1233 -> [w1278 w1283]
          tunnel: [w1279 w1281] -> w1232
          frame False {
            n247 = Enqueue Element(queue=w1278, element=T1."Powering up", error in (no error)=w1280) -> (error out=w1279:errorcluster)  [unwired: 1 in, 2 out]
          }
          frame True {
            n248 = Enqueue Element At Opposite End(queue=w1283, element=T1."Emergency", error in (no error)=w1284) -> (error out=w1281:errorcluster)  [unwired: 1 in, 2 out]
          }
        }
      }
      frame "Powering down" {
        w1323 = FALSE
        n249 = local write "Shutdown"(0.0 ("Shutdown")) -> ()
        n250 = shared-variable "RT CompactRIO Target\\Mod5\\H1 System ON"(w1323) -> ()  [unwired: 1 in, 1 out]
        n251 = shared-variable "RT CompactRIO Target\\Mod5\\K3 flase salji"(w1323) -> ()  [unwired: 1 in, 1 out]
        n252 = shared-variable "RT CompactRIO Target\\Mod5\\Y3 Retract cyl. 2"(w1323) -> ()  [unwired: 1 in, 1 out]
        n253 = Enqueue Element(queue=w1327, element=T1."Powering up", error in (no error)=w1328) -> (error out=w1325:errorcluster)  [unwired: 1 in, 2 out]
      }
    }
  }
  "error out" <- w3
